vi "50HZ pulse servo.vi"(1 "(2.5us)":u32, 2 "period (20Mhz)":u32=60606) -> (0 "50HZ pulse":bool)   [LabVIEW 2019]
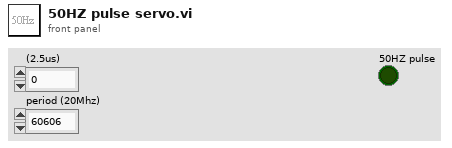
[diagram p1: front panel]
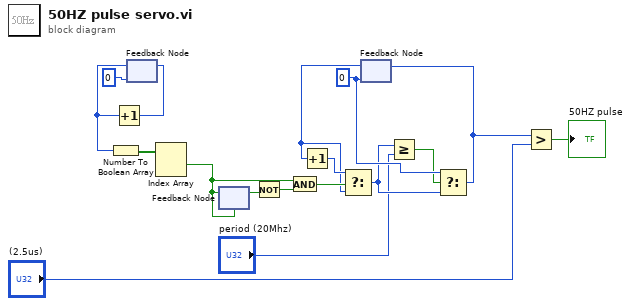
[diagram p0: block diagram]
diagram:
  w8 = u32 0
  n1 = feedback #1(u8 0) -> (w15:u8)
  n2 = Number To Boolean Array(number=w15) -> (Boolean array=w14:bool[])
  n3 = Increment(x=w15) -> (x+1=w16:u8)
  n4 = feedback-in #1(w16) -> ()
  n5 = Index Array(array=w14) -> (element #1=w2:bool)  [unwired: 2 in, 1 out]
  n6 = feedback-in #2(w2) -> ()
  n7 = feedback #2(w2) -> (w13:bool)
  n8 = Not(x=w13) -> (.not. x?=w12:bool)
  n9 = And(x=w2, y=w12) -> (x .and. y?=w11:bool)
  n10 = feedback #3(w8) -> (w9:u32)
  n11 = Increment(x=w9) -> (x+1=w10:u32)
  n12 = Select(t=w10, s=w11, f=w9) -> (s? t:f=w7:u32)
  n13 = Greater Or Equal?(x=w7, y="period (20Mhz)") -> (x >= y?=w5:bool)
  n14 = Select(t=w8, s=w5, f=w7) -> (s? t:f=w4:u32)
  n15 = feedback-in #3(w4) -> ()
  n16 = Greater?(x=w4, y="(2.5us)") -> (0:→"50HZ pulse":bool)
